vi "Test Inherit Method.vi"(8 "error in (no error)":errorcluster, 11 "Test Case Test Double Parent in":refnum<class "Test Case Test Double Parent.lvclass">) -> (0 "error out":errorcluster, 3 "Test Case Test Double Parent out":refnum<class "Test Case Test Double Parent.lvclass">)   [LabVIEW 2020, in "Test Case Test Double Parent.lvclass"]
uses:
  Test Case Test Double Parent.lvclass
  C:/git/astemes-lunit/source/API/LUnit Test Case/LUnit Test Case.lvclass
  source/API/LUnit Test Case/LUnit Test Case.lvclass/LUnit Test Case.ctl
  source/API/LUnit Test Case/Private/Append Fail Result.vi
  source/API/LUnit Test Case/Private/Append Pass Result.vi
  source/API/LUnit Test Case/Private/Run In UI.vi
  <vilib>/Utility/error.llb/Clear Errors.vi
  source/API/LUnit Test Case/LUnit Test Case.lvclass
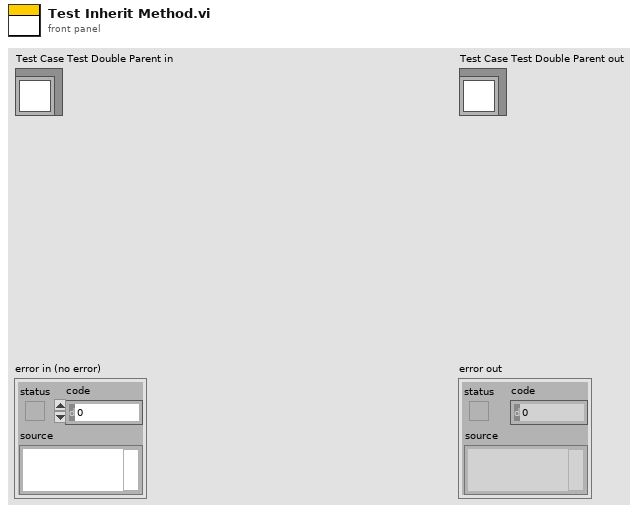
[diagram p1: front panel]
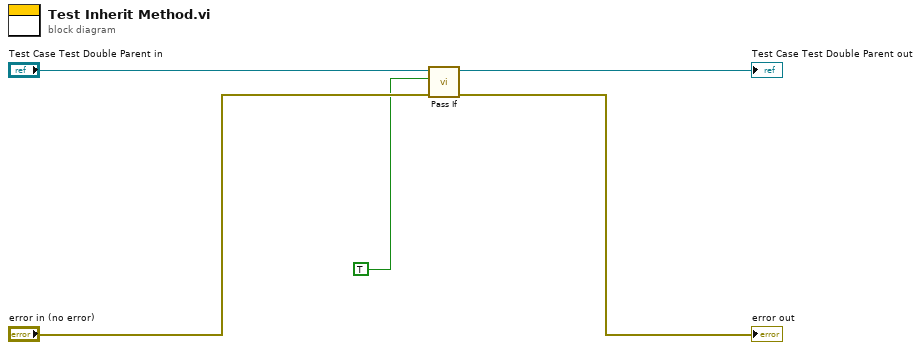
[diagram p0: block diagram]
diagram:
  n1 = call "Pass If.vi"("error in (no error)"="error in (no error)", "Pass?"=TRUE, "LUnit Test Case In"="Test Case Test Double Parent in") -> ("error out"=→"error out":errorcluster, "LUnit Test Case Out"=→"Test Case Test Double Parent out":refnum<class "Test Case Test Double Parent.lvclass">)  [unwired: 7 in]
